vi "NI Analog Input.vi"(2 "NI1":tag="Dev2", 3 "NI2":tag="Dev2") -> (16 "T1":dbl, 18 "T2":dbl, 19 "T3":dbl, 20 "T4":dbl, 21 "T5":dbl, 22 "T6":dbl, 23 "T7":dbl, 24 "T8":dbl, 25 "T9":dbl, 26 "Heater Temp":dbl, 27 "Heater Power":dbl format="%0.2f")   [LabVIEW 2017]
uses:
  <vilib>/Analysis/baseanly.llb/Mean (DBL).vi
  <vilib>/Analysis/NI_AALBase.lvlib
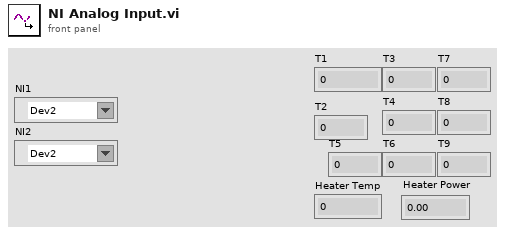
[diagram p1: front panel]
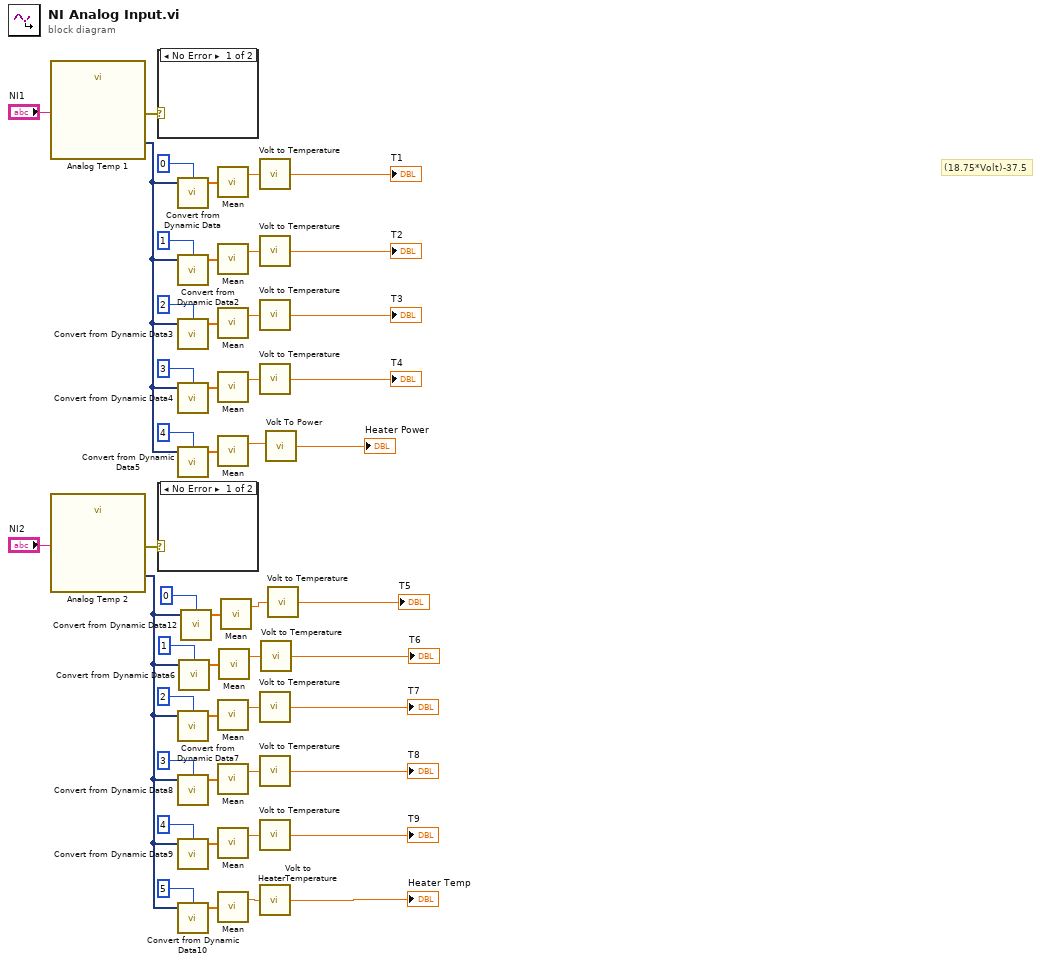
[diagram p0: block diagram]
diagram:
  # "(18.75*Volt)-37.5"
  n1 = call "Analog Temp 1"("device name"="NI1") -> ("data"=w31:dynamicdata, "error out"=w39:errorcluster)  [unwired: 16 in, 1 out]
  n2 = call "Analog Temp 2"("device name"="NI2") -> ("data"=w2:dynamicdata, "error out"=w30:errorcluster)  [unwired: 16 in, 1 out]
  n3 = case shown="No Error" w39 {
    frame No Error {
    }
    frame Error {
    }
  }
  n4 = case shown="No Error" w30 {
    frame No Error {
    }
    frame Error {
    }
  }
  n5 = call "Convert from Dynamic Data"("Dynamic Data Type"=w31, "Channel"=0) -> ("Array"=w49:dbl[])  [unwired: 2 in]
  n6 = call "Convert from Dynamic Data2"("Dynamic Data Type"=w31, "Channel"=1) -> ("Array"=w48:dbl[])  [unwired: 2 in]
  n7 = call "Convert from Dynamic Data3"("Dynamic Data Type"=w31, "Channel"=2) -> ("Array"=w45:dbl[])  [unwired: 2 in]
  n8 = call "Convert from Dynamic Data4"("Dynamic Data Type"=w31, "Channel"=3) -> ("Array"=w44:dbl[])  [unwired: 2 in]
  n9 = call "Convert from Dynamic Data5"("Dynamic Data Type"=w31, "Channel"=4) -> ("Array"=w42:dbl[])  [unwired: 2 in]
  n10 = call "Convert from Dynamic Data7"("Dynamic Data Type"=w2, "Channel"=2) -> ("Array"=w35:dbl[])  [unwired: 2 in]
  n11 = call "Convert from Dynamic Data8"("Dynamic Data Type"=w2, "Channel"=3) -> ("Array"=w32:dbl[])  [unwired: 2 in]
  n12 = call "Convert from Dynamic Data9"("Dynamic Data Type"=w2, "Channel"=4) -> ("Array"=w27:dbl[])  [unwired: 2 in]
  n13 = call "Convert from Dynamic Data10"("Dynamic Data Type"=w2, "Channel"=5) -> ("Array"=w28:dbl[])  [unwired: 2 in]
  n14 = call "Convert from Dynamic Data6"("Dynamic Data Type"=w2, "Channel"=1) -> ("Array"=w36:dbl[])  [unwired: 2 in]
  n15 = call "Convert from Dynamic Data12"("Dynamic Data Type"=w2, "Channel"=0) -> ("Array"=w4:dbl[])  [unwired: 2 in]
  n16 = call-poly <vilib>:"Mean.vi"("X"=w49) -> ("mean"=w25:dbl)  [unwired: 1 out]
  n17 = call-poly <vilib>:"Mean.vi"("X"=w48) -> ("mean"=w21:dbl)  [unwired: 1 out]
  n18 = call-poly <vilib>:"Mean.vi"("X"=w45) -> ("mean"=w20:dbl)  [unwired: 1 out]
  n19 = call-poly <vilib>:"Mean.vi"("X"=w44) -> ("mean"=w18:dbl)  [unwired: 1 out]
  n20 = call-poly <vilib>:"Mean.vi"("X"=w42) -> ("mean"=w5:dbl)  [unwired: 1 out]
  n21 = call-poly <vilib>:"Mean.vi"("X"=w35) -> ("mean"=w13:dbl)  [unwired: 1 out]
  n22 = call-poly <vilib>:"Mean.vi"("X"=w32) -> ("mean"=w11:dbl)  [unwired: 1 out]
  n23 = call-poly <vilib>:"Mean.vi"("X"=w27) -> ("mean"=w9:dbl)  [unwired: 1 out]
  n24 = call-poly <vilib>:"Mean.vi"("X"=w28) -> ("mean"=w7:dbl)  [unwired: 1 out]
  n25 = call-poly <vilib>:"Mean.vi"("X"=w36) -> ("mean"=w15:dbl)  [unwired: 1 out]
  n26 = call-poly <vilib>:"Mean.vi"("X"=w4) -> ("mean"=w1:dbl)  [unwired: 1 out]
  n27 = call "Volt to Temperature.vi"("Volt"=w25) -> ("Temperature"=→"T1":dbl)
  n28 = call "Volt to Temperature.vi"("Volt"=w21) -> ("Temperature"=→"T2":dbl)
  n29 = call "Volt to Temperature.vi"("Volt"=w20) -> ("Temperature"=→"T3":dbl)
  n30 = call "Volt to Temperature.vi"("Volt"=w18) -> ("Temperature"=→"T4":dbl)
  n31 = call "Volt to Temperature.vi"("Volt"=w13) -> ("Temperature"=→"T7":dbl)
  n32 = call "Volt to Temperature.vi"("Volt"=w11) -> ("Temperature"=→"T8":dbl)
  n33 = call "Volt to Temperature.vi"("Volt"=w9) -> ("Temperature"=→"T9":dbl)
  n34 = call "Volt to HeaterTemperature.vi"("Volt"=w7) -> ("Temperature"=→"Heater Temp":dbl)
  n35 = call "Volt to Temperature.vi"("Volt"=w15) -> ("Temperature"=→"T6":dbl)
  n36 = call "Volt To Power.vi"("Volt"=w5) -> ("Power"=→"Heater Power":dbl)
  n37 = call "Volt to Temperature.vi"("Volt"=w1) -> ("Temperature"=→"T5":dbl)
